vi "平面度检测.vi"() -> ()   [LabVIEW 2020]
panel:
  out "error out 8":errorcluster
  in  "y":bool
  out "error out 4":errorcluster
  out "element":string[](array[string])
  out "error out":errorcluster
  out "线扫通讯":bool
  out "读到的数据":string[](array[string])
  out "结果":i32
  in  "高度差返修下限":dbl format="%#_13g"
  in  "高度差返修上限":dbl format="%#_13g"
  in  "高度差上限":dbl format="%#_13g"
  in  "高度差下限":dbl format="%#_13g"
  out "error out 7":errorcluster
  out "error out 6":errorcluster
  out "error out 5":errorcluster
  in  "Numeric":i32
  out "error out 3":errorcluster
  out "error out 2":errorcluster
  in  "写入完成":bool
  out "开始采集":bool
  out "PLC通讯":bool
  out "PLC地址":string
  out "数据记录":path=path "d:/上料检测CCDNG图片"
  out "上下限":path
  out "复位":bool=TRUE
  out "日期/时间字符串":string
  out "数组":errorcluster[](array[cluster])
  in  "退出":bool
  in  "选项卡控件":enum32{"主界面", "参数设置"}(tab)
  out "完成":bool
  out "复测2":bool
  out "复测1":bool
  out "NG 2":bool
  out "OK 2":bool
  in  "测量数据":i32(listbox)
  out "NG1":bool
  out "OK1":bool
  in  "点位计算":bool
  in  "平面度内下限":dbl format="%#_13g"
  in  "平面度外上限":dbl
  in  "平面度外下限":dbl
  in  "平面度内上限":dbl
  in  "Password":string
  in  "保存":bool
  in  "平面度内复测上限":dbl format="%#_13g"
  in  "平面度外复测上限":dbl
  in  "平面度内复测下限":dbl format="%#_13g"
  in  "平面度外复测下限":dbl
  # "数据处理系统"
  # "①"
  # "②"
  # "OK范围"
  # "复测范围"
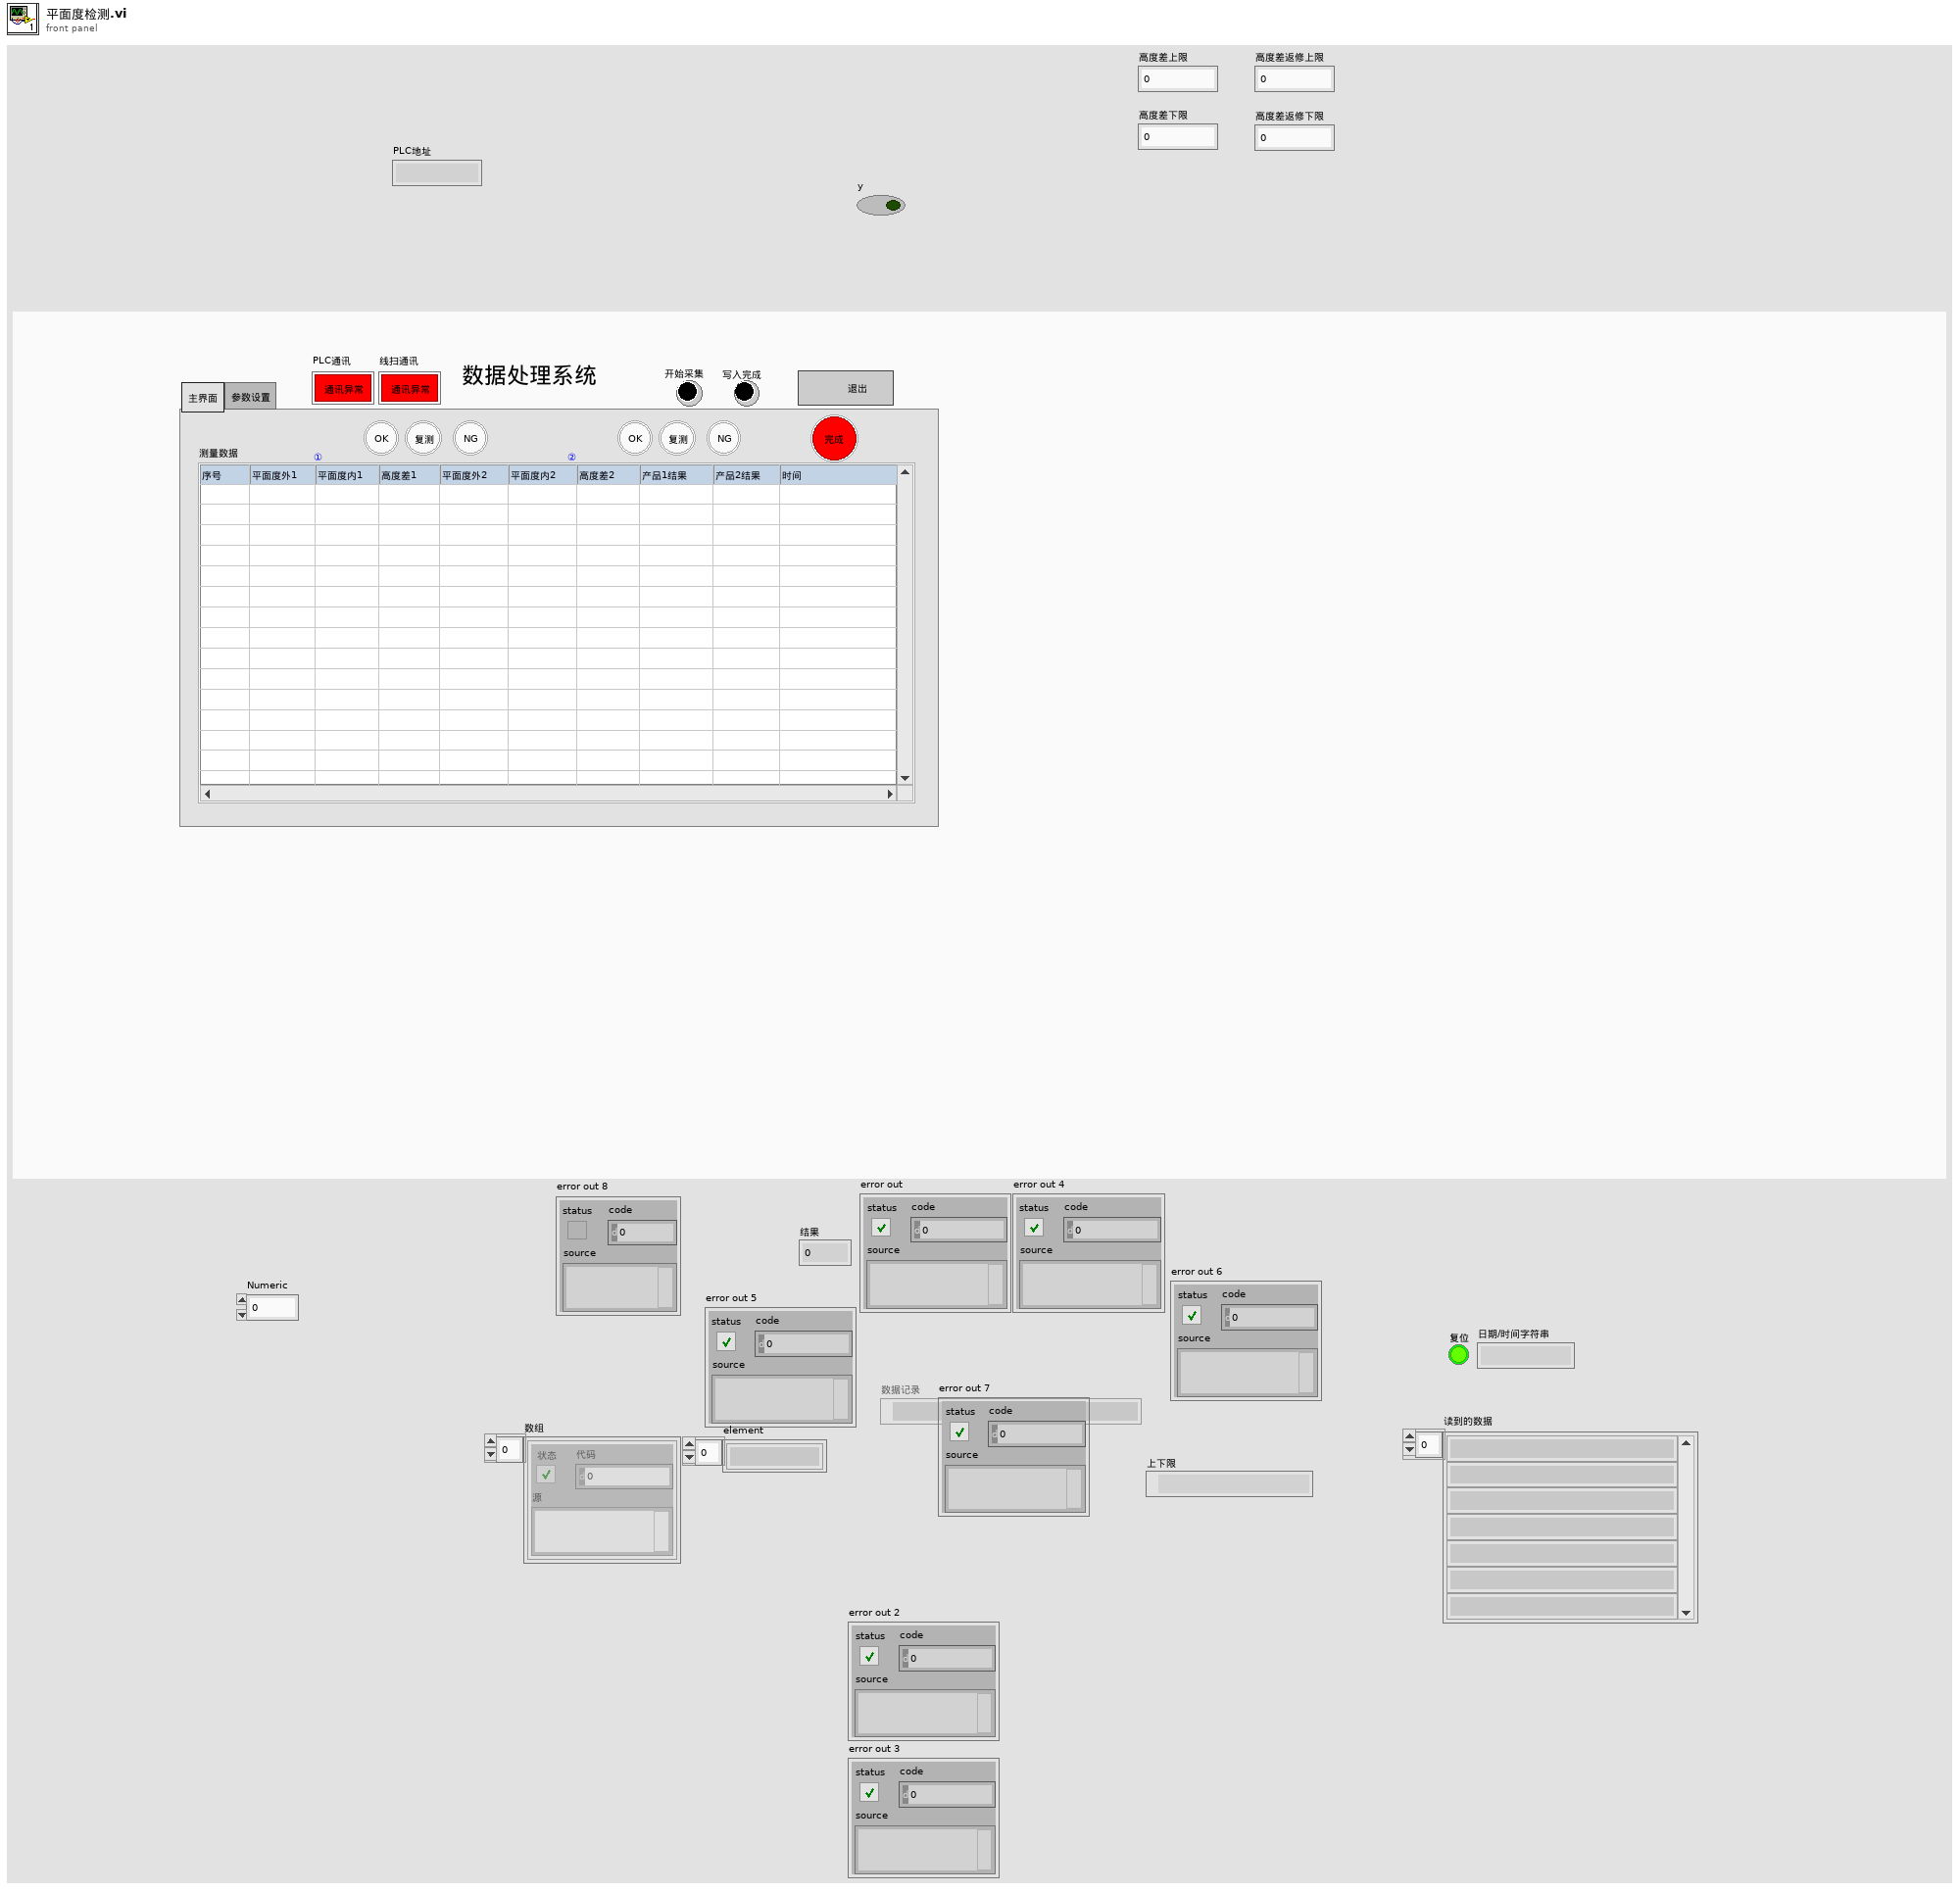
[diagram p1: front panel]
types:
  T1 = typedef "主程序枚举.ctl" = enum16{"初始化", "读取数据", "解析数据", "发送数据到PLC", "写入完成信号", "等待PLC复位", "复位信号", "关闭端口"}
  T2 = enum8{"Enabled", "Disabled", "Disabled and Grayed Out"}
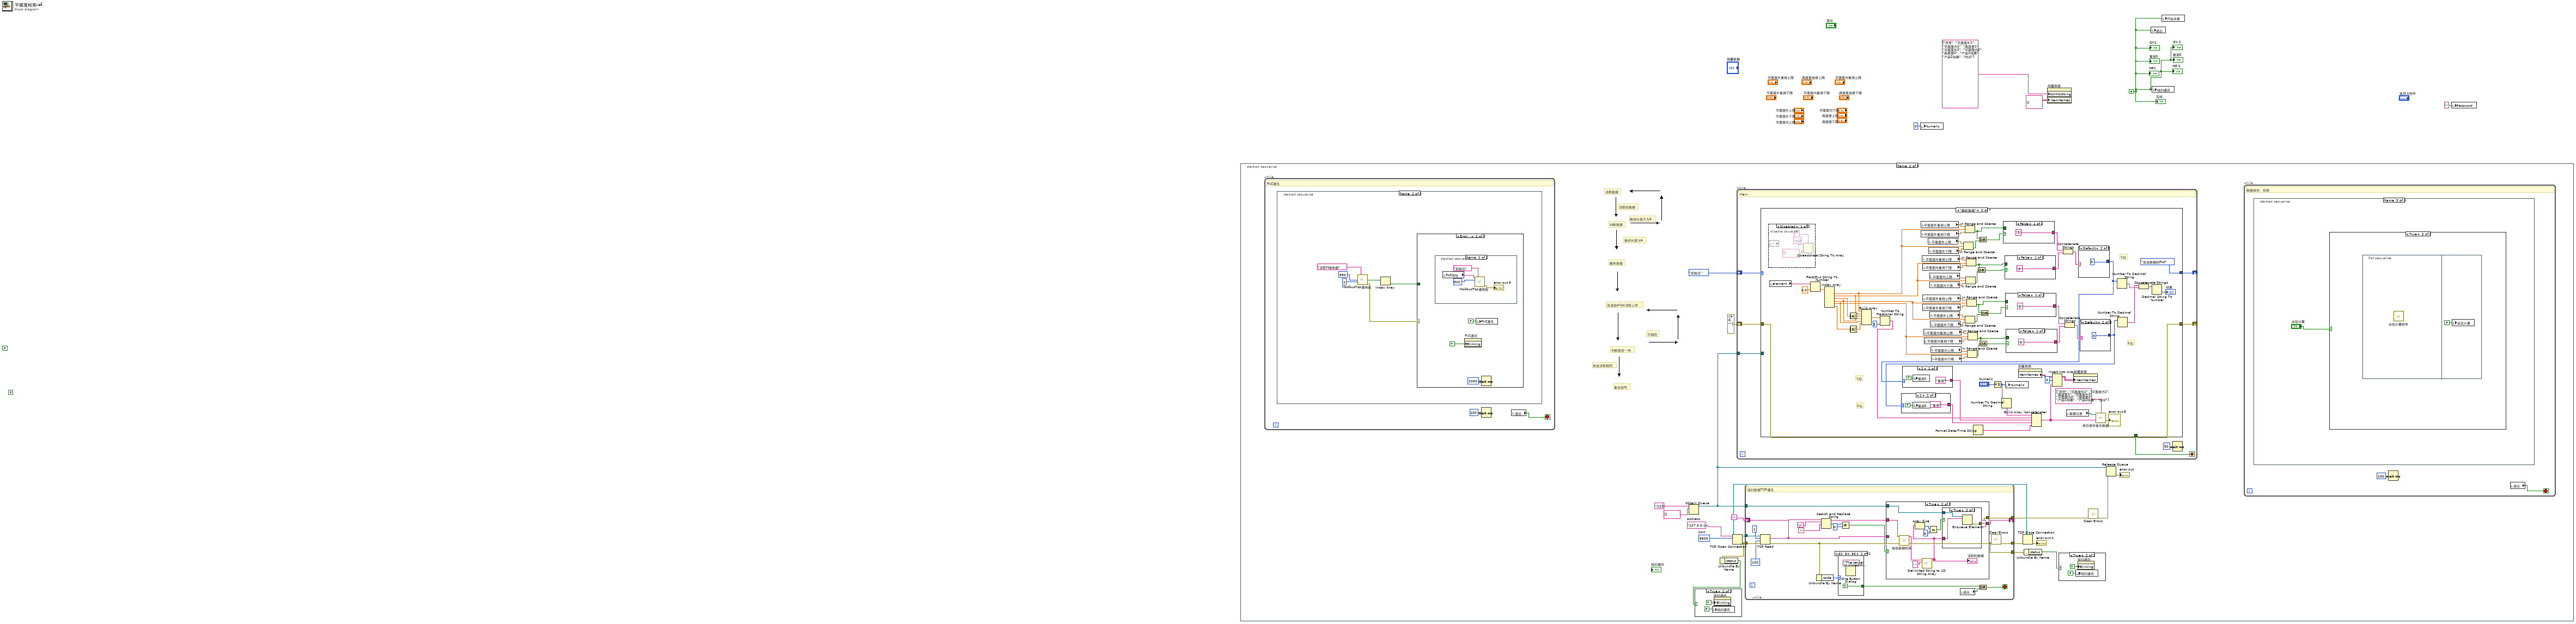
[diagram p0: block diagram]
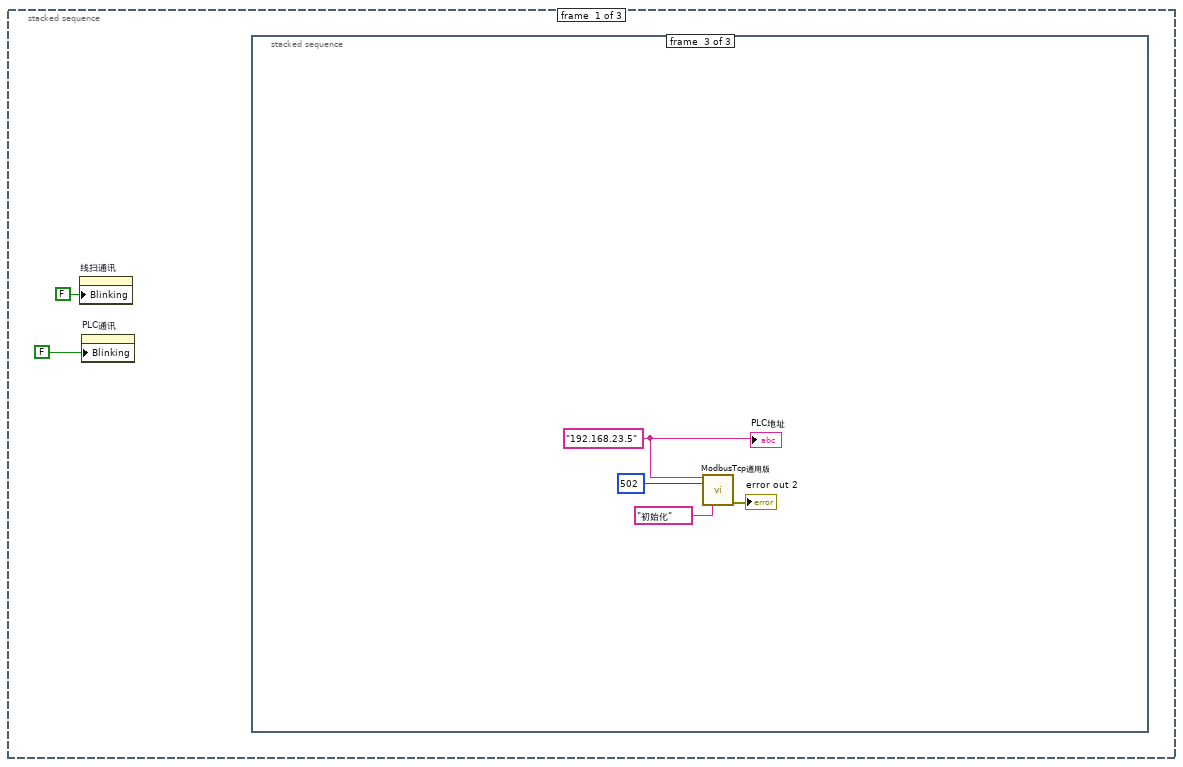
[diagram p2: hidden frame]
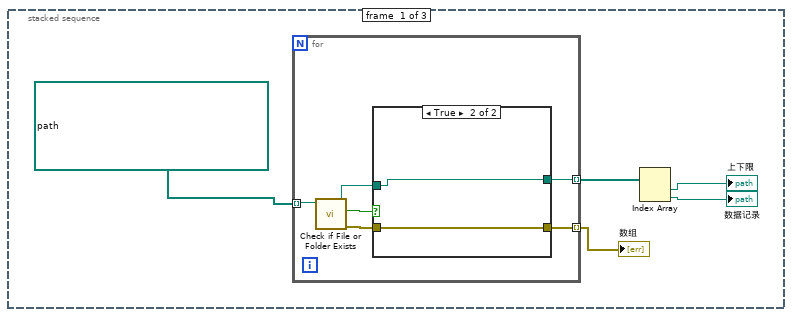
[diagram p3: hidden frame]
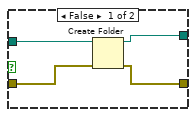
[diagram p4: hidden frame]
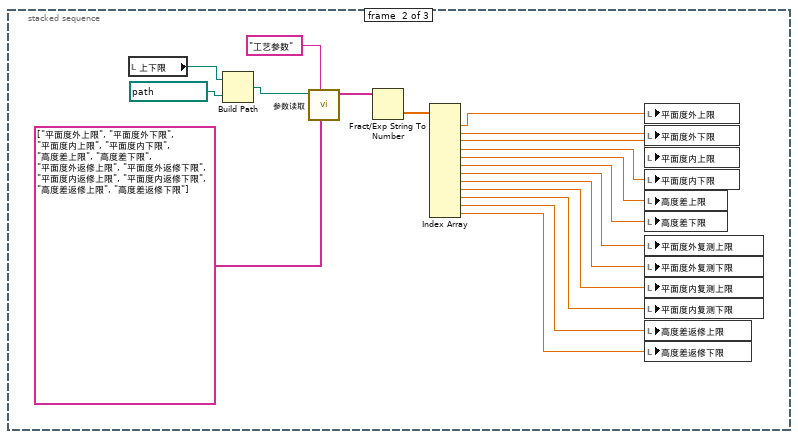
[diagram p5: hidden frame]
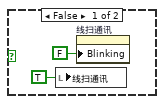
[diagram p6: hidden frame]
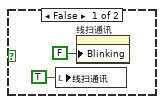
[diagram p7: hidden frame]
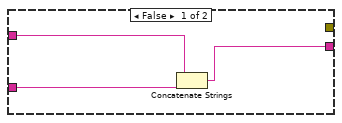
[diagram p8: hidden frame]
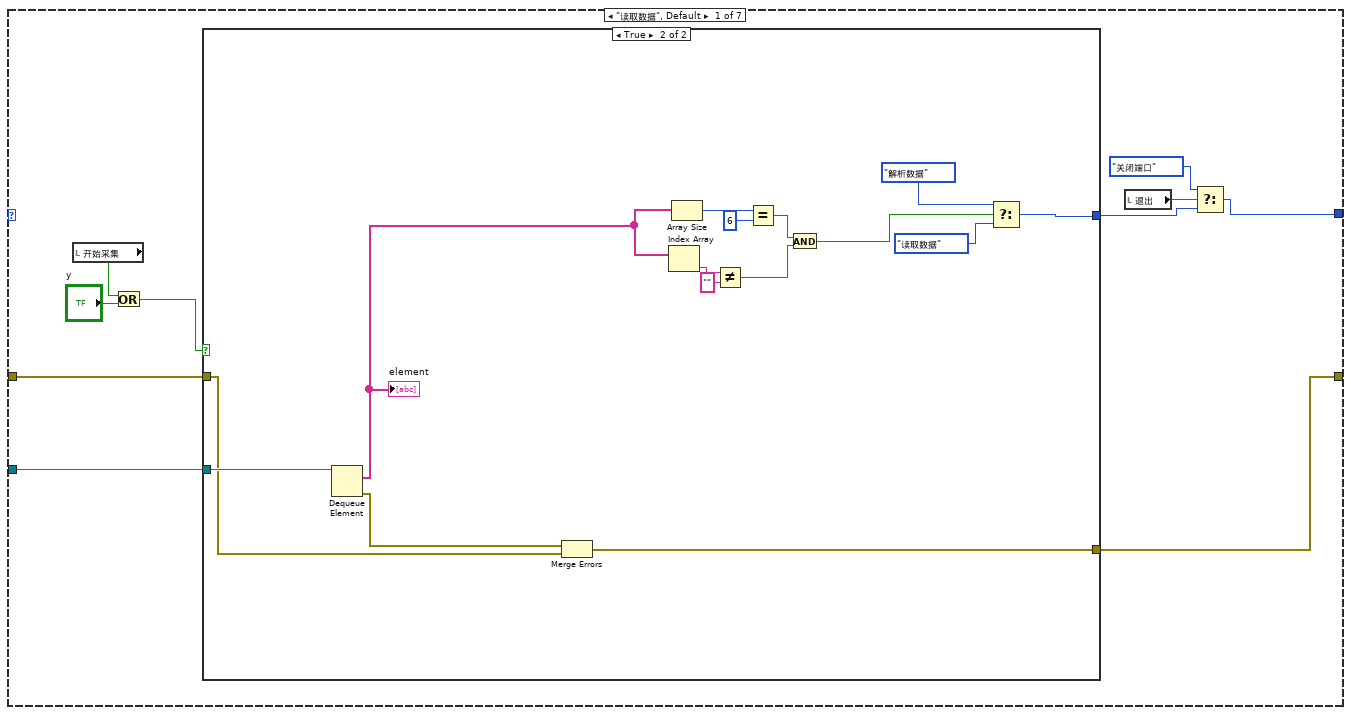
[diagram p11: hidden frame]
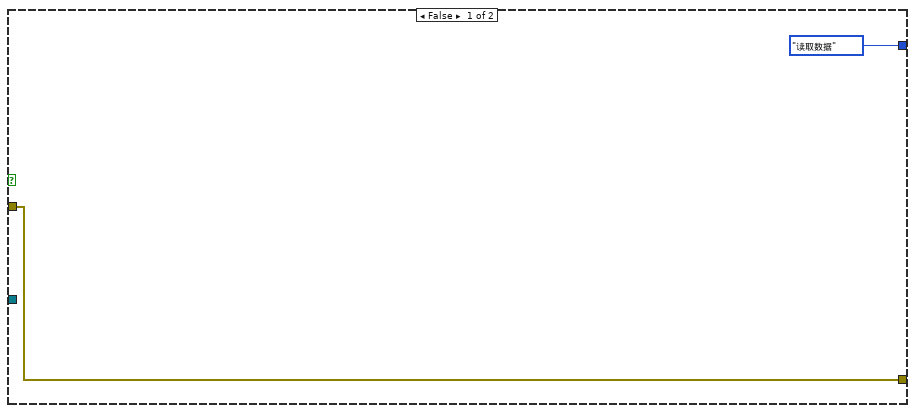
[diagram p12: hidden frame]
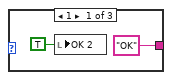
[diagram p14: hidden frame]
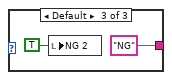
[diagram p15: hidden frame]
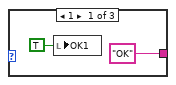
[diagram p16: hidden frame]
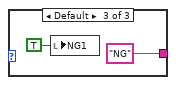
[diagram p17: hidden frame]
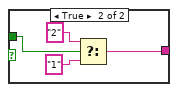
[diagram p18: hidden frame]
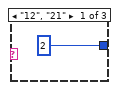
[diagram p19: hidden frame]
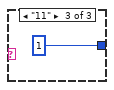
[diagram p20: hidden frame]
diagram:
  w1 = FALSE ("线扫通讯")
  (unwired) FALSE
  (unwired) FALSE
  n1 = stacked-sequence {
    frame #0 {
      n2 = property on="线扫通讯" class="Bool (strict)"("Blinking"=FALSE) -> ()  [unwired: 2 in, 2 out]
      n3 = property on="PLC通讯" class="Bool (strict)"("Blinking"=FALSE) -> ()  [unwired: 2 in, 2 out]
      n4 = stacked-sequence {
        frame #0 {
          n5 = for {
            tunnel: path[] [path "D:/上下限", path "D:/数据记录"] -> [w17] mode=indexing
            tunnel: [w14] -> w11 mode=indexing
            tunnel: [w13] -> w10 mode=indexing
            n6 = call <vilib>:"Check if File or Folder Exists.vi"("path"=w17) -> ("error out"=w15:errorcluster, "file or folder exists?"=w18:bool, "dup path"=w16:path)  [unwired: 8 in]
            n7 = case shown="True" w18 {
              tunnel: w16 -> [w22 w24]
              tunnel: w15 -> [w21 w23]
              tunnel: [w20 w24] -> w14
              tunnel: [w19 w23] -> w13
              frame False {
                n8 = Create Folder(path (use dialog)=w22, error in=w21) -> (created path=w20:path, error out=w19:errorcluster)  [unwired: 1 in, 1 out]
              }
              frame True {
              }
            }
          }
          "数组" <- w10
          n9 = Index Array(array=w11) -> (element #1=→"上下限":path, element #2=→"数据记录":path)  [unwired: 2 in]
        }
        frame #1 {
          n10 = local read "上下限"() -> (w37:path)
          n11 = Build Path(base path=w37, name or relative path=path "工艺参数.ini") -> (appended path=w38:path)
          n12 = call "参数读取.vi"("key names"=string[] ["平面度外上限", "平面度外下限", "平面度内上限", "平面度内下限", "高度差上限", "高度差下限", "平面度外返修上限", "平面度外返修下限", "平面度内返修上限", "平面度内返修下限", "高度差返修上限", "高度差返修下限"] ("键名"), "段名"="工艺参数", "configuration file path"=w38) -> ("值"=w39:string[])  [unwired: 7 in, 1 out]
          n13 = Fract/Exp String To Number(string=w39) -> (number=w40:dbl[])  [unwired: 3 in, 1 out]
          n14 = Index Array(array=w40) -> (element #1=w41:dbl, element #2=w42:dbl, element #3=w43:dbl, element #4=w34:dbl, element #5=w33:dbl, element #6=w32:dbl, element #7=w30:dbl, element #8=w29:dbl, element #9=w28:dbl, element #10=w27:dbl, element #11=w26:dbl, element #12=w25:dbl)  [unwired: 12 in]
          n15 = local write "平面度外上限"(w41) -> ()
          n16 = local write "平面度外下限"(w42) -> ()
          n17 = local write "平面度内上限"(w43) -> ()
          n18 = local write "平面度内下限"(w34) -> ()
          n19 = local write "高度差上限"(w33) -> ()
          n20 = local write "高度差下限"(w32) -> ()
          n21 = local write "平面度外复测上限"(w30) -> ()
          n22 = local write "平面度外复测下限"(w29) -> ()
          n23 = local write "平面度内复测上限"(w28) -> ()
          n24 = local write "平面度内复测下限"(w27) -> ()
          n25 = local write "高度差返修上限"(w26) -> ()
          n26 = local write "高度差返修下限"(w25) -> ()
        }
        frame #2 {
          w45 = "192.168.23.5"
          n27 = call "ModbusTcp通用版.vi"("IP Address"=w45, "操作选择"="初始化" ("Combo Box 2"), "Port"=u16 502 ("port")) -> ("error out 2"=→"error out 2":errorcluster)  [unwired: 10 in, 2 out]
          "PLC地址" <- w45
        }
      }
    }
    frame #1 {
      w58 = "127.0.0.1"  # address
      w64 = u16 8500  # port
      # "复位信号"
      # "不相同"
      # "发送读取相同"
      # "数组长度不为6"
      # "数组长度为6"
      # "读取到数据"
      # "判断是否一样"
      # "解析数据"
      # "发送给plc并读取上来"
      # "判断数据"
      # "读取数据"
      n28 = while {
        stop <- w371 stop-if-true
        # "PLC通讯"
        n29 = stacked-sequence {
          frame #0 {
            n30 = Build Array("写入完成") -> (w375:bool[])
            n31 = call "ModbusTcp通用版.vi"("操作选择"="写入多个M继电器" ("Combo Box 2"), "开始地址"=u16 991, "写继电器"=w375) -> ("error out 2"=→"error out 3":errorcluster)  [unwired: 10 in, 2 out]
          }
          frame #1 {
            n32 = call "ModbusTcp通用版.vi"("操作选择"="读取M继电器" ("Combo Box 2"), "开始地址"=u16 990, "读取个数"=u16 1) -> ("读取继电器的信号"=w380:bool[], "error out 2"=w378:errorcluster)  [unwired: 10 in, 1 out]
            n33 = Index Array(array=w380) -> (element=w379:bool)  [unwired: 1 in]
            n34 = case shown="Error .." w378 {
              tunnel: w379 -> [w386 _]
              frame No Error {
                n35 = property on="PLC通讯" class="Bool (strict)"("Blinking"=FALSE) -> ()  [unwired: 2 in, 2 out]
                "开始采集" <- w386
                "PLC通讯" <- TRUE ("PLC通讯")
              }
              frame Error {
                n36 = stacked-sequence {
                  frame #0 {
                    n37 = call "ModbusTcp通用版.vi"("操作选择"="断开") -> ("error out 2"=→"error out 6":errorcluster)  [unwired: 12 in, 2 out]
                  }
                  frame #1 {
                    n38 = local read "PLC地址"() -> (w394:string)
                    n39 = call "ModbusTcp通用版.vi"("IP Address"=w394, "操作选择"="初始化", "Port"=u16 502 ("port")) -> ("error out 2"=→"error out 5":errorcluster)  [unwired: 10 in, 2 out]
                  }
                }
                n40 = property on="PLC通讯" class="Bool (strict)"("Blinking"=TRUE) -> ()  [unwired: 2 in, 2 out]
                n41 = local write "PLC通讯"(FALSE ("PLC通讯")) -> ()
                n42 = Wait (ms)(milliseconds to wait=u32 2000 ("等待时间（毫秒）")) -> ()  [unwired: 1 out]
              }
            }
          }
        }
        n43 = Wait (ms)(milliseconds to wait=u32 100 ("等待时间（毫秒）")) -> ()  [unwired: 1 out]
        n44 = local read "退出"() -> (w371:bool)
      }
      n45 = Obtain Queue(name (unnamed)="123", element data type=string[] [] ("string array")) -> (queue out=w55:refnum<queue>)  [unwired: 3 in, 2 out]
      n46 = TCP Open Connection(address=w58, remote port or service name=w64) -> (connection ID=w63:refnum<k5>, error out=w61:errorcluster)  [unwired: 3 in]
      n47 = Unbundle By Name(w61) -> ("status"=w49:bool)
      n48 = case shown="True" w49 {
        frame False {
          n49 = local write "线扫通讯"(TRUE ("线扫通讯")) -> ()
          n50 = property on="线扫通讯" class="Bool (strict)"("Blinking"=FALSE) -> ()  [unwired: 2 in, 2 out]
        }
        frame True {
          n51 = local write "线扫通讯"(FALSE ("线扫通讯")) -> ()
          n52 = property on="线扫通讯" class="Bool (strict)"("Blinking"=TRUE) -> ()  [unwired: 2 in, 2 out]
        }
      }
      n53 = while {
        shift-right: [w116] -> _
        shift-left: errorcluster {"status"=FALSE, "code"=0, "source"=""} ("error out 2") -> [w117]
        shift-right: [w115] -> _
        shift-left: 主程序枚举."初始化" ("枚举") -> [w119]
        tunnel: w55 -> [w113]
        stop <- w114 stop-if-true
        # "Main"
        n54 = case shown="\"解析数据\"" w119 {
          tunnel: w117 -> [w129 w169 w269 w275 w277 w297 w305]
          tunnel: [w128 w169 w265 w275 w277 w297 w304] -> w116
          tunnel: [w124 主程序枚举."发送数据到PLC" ("枚举") 主程序枚举."写入完成信号" ("枚举") 主程序枚举."等待PLC复位" ("枚举") w278 w293 _] -> w115
          tunnel: [_ _ _ _ _ _ TRUE] -> w114
          tunnel: w113 -> [w123 _ _ _ _ _ _]
          frame "读取数据", Default {
            n55 = local read "开始采集"() -> (w122:bool)
            n56 = Or(x=w122, y="y") -> (x .or. y?=w120:bool)
            n57 = case shown="True" w120 {
              tunnel: w129 -> [w131 w135]
              tunnel: [主程序枚举."读取数据" ("枚举") w146] -> w125
              tunnel: [w131 w133] -> w128
              tunnel: w123 -> [_ w136]
              frame False {
              }
              frame True {
                n58 = Dequeue Element(queue=w136) -> (element=w132:string[], error out=w134:errorcluster)  [unwired: 2 in, 2 out]
                "element" <- w132
                n59 = Merge Errors(w134, w135) -> (w133:errorcluster)
                n60 = Index Array(array=w132) -> (element=w140:string)  [unwired: 1 in]
                n61 = Array Size(array=w132) -> (size(s)=w143:i32)
                n62 = Not Equal?(x=w140, y="") -> (x != y?=w137:bool)
                n63 = Equal?(x=w143, y=6) -> (x = y?=w141:bool)
                n64 = And(x=w141, y=w137) -> (x .and. y?=w138:bool)
                n65 = Select(t=主程序枚举."解析数据" ("枚举"), s=w138, f=主程序枚举."读取数据" ("枚举")) -> (s? t:f=w146:T1)
              }
            }
            n66 = local read "退出"() -> (w127:bool)
            n67 = Select(t=主程序枚举."关闭端口" ("枚举"), s=w127, f=w125) -> (s? t:f=w124:T1)
          }
          frame "解析数据" {
            # "2位"
            # "1位"
            # "2位"
            # "1位"
            n68 = disable-structure shown="Disabled" {
              frame Disabled {
                n69 = local read item#-1() -> ()  [unwired: 1 out]
                n70 = Spreadsheet String To Array(delimiter (Tab)=",", format string="%f", array type (2D Dbl)=string[] []) -> ()  [unwired: 1 in, 1 out]
              }
              frame Enabled {
              }
            }
            n71 = local read "element"() -> (w149:string[])
            n72 = Fract/Exp String To Number(string=w149, default (0 dbl)=0.0 ("default (0 DBL)")) -> (number=w206:dbl[])  [unwired: 2 in, 1 out]
            n73 = Index Array(array=w206) -> (element #1=w159:dbl, element #2=w158:dbl, element #3=w156:dbl, element #4=w155:dbl, element #5=w154:dbl, element #6=w152:dbl)  [unwired: 6 in]
            n74 = Absolute Value(x=w156) -> (abs(x)=w157:dbl)
            n75 = Absolute Value(x=w152) -> (abs(x)=w153:dbl)
            n76 = Build Array(w159, w158, w157, w155, w154, w153) -> (w151:dbl[])
            n77 = Number To Fractional String(number=w151, precision (6)=i16 3) -> (F-format string=w148:string[])  [unwired: 2 in]
            n78 = local read "平面度外复测上限"() -> (w205:dbl)
            n79 = local read "平面度外复测下限"() -> (w204:dbl)
            n80 = local read "平面度内复测上限"() -> (w203:dbl)
            n81 = local read "平面度内复测下限"() -> (w202:dbl)
            n82 = local read "平面度外复测上限"() -> (w174:dbl)
            n83 = local read "平面度外复测下限"() -> (w175:dbl)
            n84 = local read "平面度内复测上限"() -> (w176:dbl)
            n85 = local read "平面度内复测下限"() -> (w177:dbl)
            n86 = local read "平面度外上限"() -> (w200:dbl)
            n87 = local read "平面度外下限"() -> (w201:dbl)
            n88 = local read "平面度内上限"() -> (w196:dbl)
            n89 = local read "平面度内下限"() -> (w161:dbl)
            n90 = local read "平面度外上限"() -> (w179:dbl)
            n91 = local read "平面度外下限"() -> (w178:dbl)
            n92 = local read "平面度内上限"() -> (w183:dbl)
            n93 = local read "平面度内下限"() -> (w162:dbl)
            n94 = In Range and Coerce(upper limit=w200, x=w159, lower limit=w201) -> (In Range?=w199:bool)  [unwired: 1 out]
            n95 = In Range and Coerce(upper limit=w205, x=w159, lower limit=w204) -> (In Range?=w197:bool)  [unwired: 1 out]
            n96 = In Range and Coerce(upper limit=w179, x=w155, lower limit=w178) -> (In Range?=w180:bool)  [unwired: 1 out]
            n97 = In Range and Coerce(upper limit=w196, x=w158, lower limit=w161) -> (In Range?=w195:bool)  [unwired: 1 out]
            n98 = In Range and Coerce(upper limit=w203, x=w158, lower limit=w202) -> (In Range?=w193:bool)  [unwired: 1 out]
            n99 = In Range and Coerce(upper limit=w174, x=w155, lower limit=w175) -> (In Range?=w182:bool)  [unwired: 1 out]
            n100 = In Range and Coerce(upper limit=w183, x=w154, lower limit=w162) -> (In Range?=w184:bool)  [unwired: 1 out]
            n101 = In Range and Coerce(upper limit=w176, x=w154, lower limit=w177) -> (In Range?=w186:bool)  [unwired: 1 out]
            n102 = Format Date/Time String() -> (date/time string=w212:string)  [unwired: 3 in]
            n103 = Or(x=w193, y=w195) -> (x .or. y?=w194:bool)
            n104 = Or(x=w197, y=w199) -> (x .or. y?=w198:bool)
            n105 = Or(x=w186, y=w184) -> (x .or. y?=w185:bool)
            n106 = Or(x=w182, y=w180) -> (x .or. y?=w181:bool)
            n107 = Increment(x="Numeric") -> (x+1=w210:i32)
            n108 = Number To Decimal String(number=w210) -> (decimal integer string=w211:string)  [unwired: 1 in]
            n109 = case shown="False" w198 {
              tunnel: w197 -> [_ w256]
              tunnel: ["3" w253] -> w192
              frame False {
              }
              frame True {
                n110 = Select(t="2", s=w256, f="1") -> (s? t:f=w253:string)
              }
            }
            n111 = case shown="False" w194 {
              tunnel: w193 -> [_ w248]
              tunnel: ["3" w245] -> w191
              frame False {
              }
              frame True {
                n112 = Select(t="2", s=w248, f="1") -> (s? t:f=w245:string)
              }
            }
            n113 = case shown="False" w181 {
              tunnel: w182 -> [_ w243]
              tunnel: ["3" w240] -> w187
              frame False {
              }
              frame True {
                n114 = Select(t="2", s=w243, f="1") -> (s? t:f=w240:string)
              }
            }
            n115 = local write "Numeric"(w210) -> ()
            n116 = case shown="False" w185 {
              tunnel: w186 -> [_ w235]
              tunnel: ["3" w232] -> w188
              frame False {
              }
              frame True {
                n117 = Select(t="2", s=w235, f="1") -> (s? t:f=w232:string)
              }
            }
            n118 = property on="测量数据" class="MCListbox (strict)"() -> ("ItemNames"=w213:string[][])  [unwired: 2 in, 2 out]
            n119 = Concatenate Strings(w192, w191) -> (w190:string)
            n120 = Concatenate Strings(w187, w188) -> (w189:string)
            n121 = local read "数据记录"() -> (w208:path)
            n122 = case shown="Default" w190 {
              tunnel: [2 3 1] -> w168
              frame "12", "21" {
              }
              frame Default {
              }
              frame "11" {
              }
            }
            n123 = case shown="2" w168 {
              tunnel: ["OK" "复测" "NG"] -> w173
              frame 1 {
                n124 = local write "OK1"(TRUE ("OK1")) -> ()
              }
              frame 2 {
                n125 = local write "复测1"(TRUE ("返修1")) -> ()
              }
              frame Default {
                n126 = local write "NG1"(TRUE ("NG1")) -> ()
              }
            }
            n127 = case shown="Default" w189 {
              tunnel: [2 3 1] -> w166
              frame "12", "21" {
              }
              frame Default {
              }
              frame "11" {
              }
            }
            n128 = case shown="2" w166 {
              tunnel: ["OK" "复测" "NG"] -> w172
              frame 1 {
                n129 = local write "OK 2"(TRUE ("OK 2")) -> ()
              }
              frame 2 {
                n130 = local write "复测2"(TRUE ("返修2")) -> ()
              }
              frame Default {
                n131 = local write "NG 2"(TRUE ("NG 2")) -> ()
              }
            }
            n132 = Build Array (concatenate)(w211, w148, w173, w172, w212) -> (w214:string[])
            n133 = Insert Into Array(array=w213, index (row)=0, new element=w214) -> (w215:string[][])  [unwired: 1 in]
            n134 = property on="测量数据" class="MCListbox (strict)"("ItemNames"=w215) -> ()  [unwired: 2 in, 2 out]
            n135 = call "按日保存每天数据.vi"("列首"=string[] ["序号", "平面度外1", "平面度内1", "高度差1", "平面度外2", "平面度内2", "高度差2", "产品1结果", "产品2结果", "时间"], "保存内容"=w214, "保存路径"=w208) -> ("error out 3"=→"error out 8":errorcluster)  [unwired: 1 in, 1 out]
            n136 = Number To Decimal String(number=w168) -> (decimal integer string=w167:string)  [unwired: 1 in]
            n137 = Number To Decimal String(number=w166) -> (decimal integer string=w165:string)  [unwired: 1 in]
            n138 = Concatenate Strings(w165, w167) -> (w164:string)
            n139 = Decimal String To Number(string=w164) -> (number=→"结果":i32)  [unwired: 2 in, 1 out]
          }
          frame "发送数据到PLC" {
            n140 = local read "结果"() -> (w268:i32)
            n141 = Build Array(w268) -> (w267:i32[])
            n142 = call "ModbusTcp通用版.vi"("操作选择"="写入单个D寄存器", "开始地址"=u16 990, "写入数组"=w267, "error in"=w269) -> ("error out 2"=w266:errorcluster)  [unwired: 9 in, 2 out]
            n143 = call "ModbusTcp通用版.vi"("操作选择"="16位读取D寄存器", "开始地址"=u16 990, "读取个数"=u16 1, "error in"=w266) -> ("读取的数据"=w260:i32[], "error out 2"=w265:errorcluster)  [unwired: 9 in, 1 out]
            n144 = local read "结果"() -> (w258:i32)
            n145 = Index Array(array=w260) -> (element=w259:i32)  [unwired: 1 in]
            n146 = Equal?(x=w259, y=w258) -> (x = y?=w257:bool)
            n147 = case shown="True" w257 {
              frame False {
                n148 = local write "完成"(FALSE ("完成")) -> ()
              }
              frame True {
                n149 = local write "完成"(TRUE ("完成")) -> ()
              }
            }
          }
          frame "写入完成信号" {
            n150 = local write "写入完成"(TRUE ("写入数据完成 M991")) -> ()
          }
          frame "等待PLC复位" {
            n151 = local read "开始采集"() -> (w283:bool)
            n152 = local read "退出"() -> (w282:bool)
            n153 = Compound Arithmetic op=OR ("复合运算")(invert w283, w282) -> (w281:bool)
            n154 = Select(t=主程序枚举."复位信号" ("枚举"), s=w281, f=主程序枚举."等待PLC复位" ("枚举")) -> (s? t:f=w278:T1)
          }
          frame "复位信号" {
            w286 = 200 ("y")
            w291 = FALSE ("写入数据完成 M100")
            n155 = property on="测量数据" class="MCListbox (strict)"() -> ("ItemNames"=w285:string[][])  [unwired: 2 in, 2 out]
            n156 = local write "读到的数据"(string[] [] ("string array 2")) -> ()
            n157 = Index Array(array=w285, index (col)=0 ("禁用的索引 (列)")) -> (element=w290:string[])  [unwired: 1 in]
            n158 = Array Size(array=w290) -> (size(s)=w288:i32)
            n159 = Greater Or Equal?(x=w288, y=w286) -> (x >= y?=w287:bool)
            n160 = case shown="True" w287 {
              tunnel: w285 -> [w298 w302]
              tunnel: w286 -> [_ w301]
              tunnel: [w298 w299] -> w284
              frame False {
              }
              frame True {
                n161 = Decrement(x=w301) -> (x-1=w300:i32)
                n162 = Delete From Array "Delete From Array"(array=w302, index (row)=w300) -> (array with subset deleted=w299:string[][])  [unwired: 2 in, 1 out]
              }
            }
            n163 = local write "NG 2"(w291) -> ()
            n164 = local write "OK 2"(w291) -> ()
            n165 = local write "复测2"(w291) -> ()
            n166 = local write "复测1"(w291) -> ()
            n167 = local write "NG1"(w291) -> ()
            n168 = local write "OK1"(w291) -> ()
            n169 = local write "写入完成"(w291) -> ()
            n170 = local write "写入完成"(w291) -> ()
            n171 = property on="测量数据" class="MCListbox (strict)"("ItemNames"=w284) -> ()  [unwired: 2 in, 2 out]
            n172 = local read "退出"() -> (w296:bool)
            n173 = Select(t=主程序枚举."关闭端口" ("枚举"), s=w296, f=主程序枚举."读取数据" ("枚举")) -> (s? t:f=w293:T1)
          }
          frame "关闭端口" {
            n174 = call "ModbusTcp通用版.vi"("操作选择"="断开", "error in"=w305) -> ("error out 2"=w304:errorcluster)  [unwired: 11 in, 2 out]
          }
        }
        n175 = Wait (ms)(milliseconds to wait=u32 50 ("等待时间（毫秒）")) -> ()  [unwired: 1 out]
      }
      n176 = while {
        tunnel: w61 -> [w92]
        tunnel: w63 -> [w93]
        tunnel: [w88] -> w60
        tunnel: [w84] -> w59
        tunnel: w55 -> [w83]
        tunnel: [w82] -> w56
        shift-right: [w74] -> _
        shift-left: "" -> [w75]
        stop <- w85 stop-if-true
        # "线扫数据TCP通讯"
        n177 = TCP Read(connection ID=w93, bytes to read=1, error in (no error)=w92, 9:100 ("timeout ms (25000)")) -> (data out=w76:string, error out=w84:errorcluster)  [unwired: 1 in, 1 out]
        n178 = Unbundle By Name(w84) -> ("code"=w89:i32)
        n179 = Search and Replace String(input string=w76, search string="\r", replace string="") -> (number of replacements=w81:i32)  [unwired: 5 in, 3 out]
        n180 = case shown="62, 64, 66" w89 {
          tunnel: [FALSE TRUE] -> w87
          frame Default {
          }
          frame 62, 64, 66 {
            n181 = One Button Dialog(message="The server VI closed the connection." ("Server Closed 2")) -> ()  [unwired: 1 in, 1 out]
          }
        }
        n182 = Not Equal?(x=w81, y=0) -> (x != y?=w79:bool)
        n183 = case shown="True" w79 {
          tunnel: w76 -> [w95 _]
          tunnel: w83 -> [_ w105]
          tunnel: [_ w102] -> w82
          tunnel: w75 -> [w96 w98]
          tunnel: [w94 ""] -> w74
          frame False {
            n184 = Concatenate Strings(w96, w95) -> (w94:string)
          }
          frame True {
            n185 = call "接收数据防呆.vi"("重复数据输入"=w98) -> ("数据输出"=w104:string)  [unwired: 10 in]
            n186 = call <vilib>:"Delimited String to 1D String Array.vi"("delimiter"=",", "delimited string"=w104) -> ("string array"=w100:string[])  [unwired: 9 in]
            "读到的数据" <- w100
            n187 = Array Size(array=w100) -> (size(s)=w101:i32)
            n188 = Equal?(x=w101, y=6) -> (x = y?=w99:bool)
            n189 = case shown="True" w99 {
              tunnel: w105 -> [_ w109]
              tunnel: w100 -> [_ w107]
              tunnel: [_ w108] -> w102
              frame False {
              }
              frame True {
                n190 = Enqueue Element(queue=w109, element=w107) -> (error out=w108:errorcluster)  [unwired: 2 in, 2 out]
              }
            }
          }
        }
        n191 = local read "退出"() -> (w86:bool)
        n192 = Or(x=w87, y=w86) -> (x .or. y?=w85:bool)
        n193 = call <vilib>:"Clear Errors.vi"("error in (no error)"=w84) -> ("error out"=w88:errorcluster)  [unwired: 5 in, 1 out]
      }
      n194 = TCP Close Connection(connection ID=w63, error in (no error)=w60) -> (error out=→"error out 4":errorcluster)  [unwired: 1 in, 1 out]
      n195 = Unbundle By Name(w59) -> ("status"=w48:bool)
      n196 = case shown="True" w48 {
        frame False {
          n197 = local write "线扫通讯"(TRUE ("线扫通讯")) -> ()
          n198 = property on="线扫通讯" class="Bool (strict)"("Blinking"=FALSE) -> ()  [unwired: 2 in, 2 out]
        }
        frame True {
          n199 = local write "线扫通讯"(FALSE ("线扫通讯")) -> ()
          n200 = property on="线扫通讯" class="Bool (strict)"("Blinking"=TRUE) -> ()  [unwired: 2 in, 2 out]
        }
      }
      n201 = call <vilib>:"Clear Errors.vi"("error in (no error)"=w56) -> ("error out"=w54:errorcluster)  [unwired: 5 in, 1 out]
      n202 = Release Queue(queue=w55, error in (no error)=w54) -> (error out=→"error out":errorcluster)  [unwired: 1 in, 2 out]
      n203 = while {
        stop <- w307 stop-if-true
        # "数据保存、权限"
        n204 = stacked-sequence {
          frame #0 {
            n205 = First Call?() -> (First Call?: T/F=w309:bool)
            n206 = local read "复位"() -> (w310:bool)
            n207 = Or(x=w310, y=w309) -> (x .or. y?=w311:bool)
            n208 = case shown="True" w311 {
              frame False {
                n209 = local read "日期/时间字符串"() -> (w312:string)
                n210 = Format Date/Time String(time format string (%c)="%M" ("时间格式字符串(%c)")) -> (date/time string=w319:string)  [unwired: 2 in]
                n211 = Fract/Exp String To Number(string=w319) -> (number=w317:dbl)  [unwired: 3 in, 1 out]
                n212 = Fract/Exp String To Number(string=w312) -> (number=w318:dbl)  [unwired: 3 in, 1 out]
                n213 = Subtract(x=w318, y=w317) -> (x-y=w316:dbl)
                n214 = Absolute Value(x=w316) -> (abs(x)=w313:dbl)
                n215 = Greater Or Equal?(x=w313, y=5.0) -> (x >= y?=w315:bool)
                n216 = case shown="False" w315 {
                  frame False {
                  }
                  frame True {
                    n217 = local write "复位"(TRUE ("复位")) -> ()
                  }
                }
              }
              frame True {
                n218 = Get Date/Time String() -> (date string=w331:string, time string=w338:string)  [unwired: 3 in]
                n219 = String Subset(string=w338, length (rest)=2 ("长度（剩余）")) -> ()  [unwired: 1 in, 1 out]
                n220 = String Subset(string=w338, offset (0)=3 ("偏移量(0)"), length (rest)=2 ("长度（剩余）")) -> ()  [unwired: 1 out]
                n221 = String Subset(string=w331, length (rest)=4 ("length (rest)")) -> (substring=w330:string)  [unwired: 1 in]
                n222 = String Subset(string=w331, offset (0)=5, length (rest)=2 ("length (rest)")) -> (substring=w329:string)
                n223 = String Subset(string=w331, offset (0)=8, length (rest)=2 ("length (rest)")) -> (substring=w328:string)
                n224 = Concatenate Strings(w330, w329, w328) -> (w341:string)
                n225 = Equal?(x="Password", y="admin") -> (x = y?=w326:bool)
                n226 = Equal?(x=w341, y="Password") -> (x = y?=w327:bool)
                n227 = Or(x=w327, y=w326) -> (x .or. y?=w323:bool)
                n228 = case shown="True" w323 {
                  tunnel: [T2."Disabled and Grayed Out" ("禁用") T2."Enabled" ("禁用")] -> w322
                  frame False {
                  }
                  frame True {
                    n229 = Format Date/Time String(time format string (%c)="%M" ("时间格式字符串(%c)")) -> (date/time string=→"日期/时间字符串":string)  [unwired: 2 in]
                    n230 = local write "Password"("" ("Password")) -> ()
                    "复位" <- FALSE
                  }
                }
                n231 = property on="高度差返修下限" class="DigNum (strict)"("DisabledEnum"=w322) -> ()  [unwired: 2 in, 2 out]
                n232 = property on="高度差返修上限" class="DigNum (strict)"("DisabledEnum"=w322) -> ()  [unwired: 2 in, 2 out]
                n233 = property on="平面度外复测下限" class="DigNum (strict)"("DisabledEnum"=w322) -> ()  [unwired: 2 in, 2 out]
                n234 = property on="平面度外复测上限" class="DigNum (strict)"("DisabledEnum"=w322) -> ()  [unwired: 2 in, 2 out]
                n235 = property on="平面度内复测上限" class="DigNum (strict)"("DisabledEnum"=w322) -> ()  [unwired: 2 in, 2 out]
                n236 = property on="平面度内复测下限" class="DigNum (strict)"("DisabledEnum"=w322) -> ()  [unwired: 2 in, 2 out]
                n237 = property on="保存" class="Bool (strict)"("DisabledEnum"=w322) -> ()  [unwired: 2 in, 2 out]
                n238 = property on="点位计算" class="Bool (strict)"("DisabledEnum"=w322) -> ()  [unwired: 2 in, 2 out]
                n239 = property on="平面度外上限" class="DigNum (strict)"("DisabledEnum"=w322) -> ()  [unwired: 2 in, 2 out]
                n240 = property on="平面度内上限" class="DigNum (strict)"("DisabledEnum"=w322) -> ()  [unwired: 2 in, 2 out]
                n241 = property on="高度差下限" class="DigNum (strict)"("DisabledEnum"=w322) -> ()  [unwired: 2 in, 2 out]
                n242 = property on="平面度外下限" class="DigNum (strict)"("DisabledEnum"=w322) -> ()  [unwired: 2 in, 2 out]
                n243 = property on="平面度内下限" class="DigNum (strict)"("DisabledEnum"=w322) -> ()  [unwired: 2 in, 2 out]
                n244 = property on="高度差上限" class="DigNum (strict)"("DisabledEnum"=w322) -> ()  [unwired: 2 in, 2 out]
              }
            }
          }
          frame #1 {
            n245 = case shown="True" "保存" {
              frame False {
              }
              frame True {
                n246 = stacked-sequence {
                  frame #0 {
                    n247 = local read "平面度外复测上限"() -> (w354:dbl)
                    n248 = local read "平面度外复测下限"() -> (w353:dbl)
                    n249 = local read "平面度内复测上限"() -> (w352:dbl)
                    n250 = local read "平面度内复测下限"() -> (w351:dbl)
                    n251 = local read "高度差返修上限"() -> (w350:dbl)
                    n252 = local read "高度差返修下限"() -> (w349:dbl)
                    n253 = local read "平面度外上限"() -> (w363:dbl)
                    n254 = local read "平面度外下限"() -> (w362:dbl)
                    n255 = local read "平面度内上限"() -> (w361:dbl)
                    n256 = local read "平面度内下限"() -> (w358:dbl)
                    n257 = local read "高度差上限"() -> (w357:dbl)
                    n258 = local read "高度差下限"() -> (w356:dbl)
                    n259 = local read "上下限"() -> (w367:path)
                    n260 = Build Array(w363, w362, w361, w358, w357, w356, w354, w353, w352, w351, w350, w349) -> (w360:dbl[])
                    n261 = Build Path(base path=w367, name or relative path=path "工艺参数.ini") -> (appended path=w365:path)
                    n262 = Number To Fractional String(number=w360) -> (F-format string=w359:string[])  [unwired: 3 in]
                    n263 = call "参数保存.vi"("段名"="工艺参数", "值"=w359, "键"=string[] ["平面度外上限", "平面度外下限", "平面度内上限", "平面度内下限", "高度差上限", "高度差下限", "平面度外返修上限", "平面度外返修下限", "平面度内返修上限", "平面度内返修下限", "高度差返修上限", "高度差返修下限"] ("键名"), "configuration file path"=w365) -> ()  [unwired: 8 in]
                  }
                  frame #1 {
                    n264 = local write "保存"(FALSE ("保存")) -> ()
                  }
                }
              }
            }
          }
          frame #2 {
            n265 = case shown="True" "点位计算" {
              frame False {
              }
              frame True {
                n266 = flat-sequence {
                  frame #0 {
                    n267 = call "点位计算软件.vi"() -> ()  [unwired: 12 in]
                  }
                  frame #1 {
                    n268 = local write "点位计算"(FALSE ("点位计算")) -> ()
                  }
                }
              }
            }
          }
        }
        n269 = Wait (ms)(milliseconds to wait=u32 200) -> ()  [unwired: 1 out]
        n270 = local read "退出"() -> (w307:bool)
      }
    }
    frame #2 {
      n271 = flat-sequence {
        frame #0 {
          n272 = call "ModbusTcp通用版.vi"("操作选择"="断开") -> ("error out 2"=→"error out 7":errorcluster)  [unwired: 12 in, 2 out]
        }
        frame #1 {
          n273 = Quit LabVIEW(quit? (T)=TRUE ("退出？(T)")) -> ()
        }
      }
    }
  }
  n274 = local write "Numeric"(0 ("Numeric")) -> ()
  n275 = property on="测量数据" class="MCListbox (strict)"("ColHdrString"=string[] ["序号", "平面度外1", "平面度内1", "高度差1", "平面度外2", "平面度内2", "高度差2", "产品1结果", "产品2结果", "时间"] ("列首"), "ItemNames"=string[][] [] ("Item Names")) -> ()  [unwired: 2 in, 2 out]
  n276 = local write "退出"(w1) -> ()
  n277 = local write "线扫通讯"(w1) -> ()
  n278 = local write "开始采集"(w1) -> ()
  n279 = local write "Password"("" ("Password")) -> ()
  "OK 2" <- w1
  "NG 2" <- w1
  "复测2" <- w1
  "OK1" <- w1
  "NG1" <- w1
  "复测1" <- w1
  "完成" <- w1
